vi "IBArray.vi"(11 "Current":sgl[](array[numeric])) -> (3 "Array":dbl[](array[numeric]))   [LabVIEW 2013]
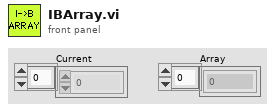
[diagram p1: front panel]
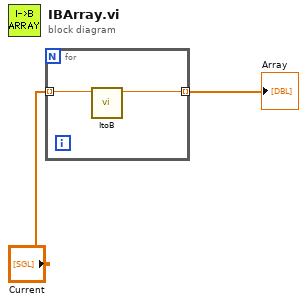
[diagram p0: block diagram]
diagram:
  n1 = for {
    tunnel: "Current" -> [w4] mode=indexing
    tunnel: [w3] -> w2 mode=indexing
    n2 = call "ItoB.vi"("Current"=w4) -> ("Field"=w3:dbl)  [unwired: 10 in]
  }
  "Array" <- w2
